vi "Configure Channel (DI Normal).vi"(0 "VISA resource name":refnum<visa-resource-name>, 5 "Channel (0001)":string="0001", 7 "Enable Channel (True)":bool=TRUE, 9 "Span":T1={"Lower Span (0)"=0, "Upper Span (1)"=1} {"Upper Span (1)" min=-99999 max=99999 step=1; "Lower Span (0)" min=-99999 max=99999 step=1}, 11 "error in (no error)":errorcluster) -> (4 "VISA resource name out":refnum<visa-resource-name>, 6 "Channel":string, 15 "error out":errorcluster)   [LabVIEW 2020, in "Yokogawa GX Series.lvlib"]
doc: "Sets the input range of DI channels.\n\nCommand: SRangeDI"
uses:
  <instrlib>/Yokogawa GX Series/Yokogawa GX Series.lvlib
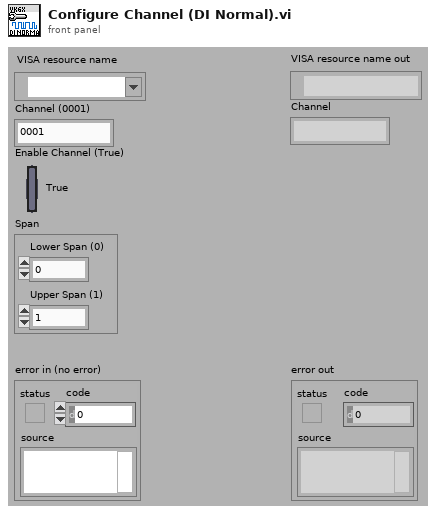
[diagram p1: front panel]
types:
  T1 = cluster{"Lower Span (0)":i32, "Upper Span (1)":i32}
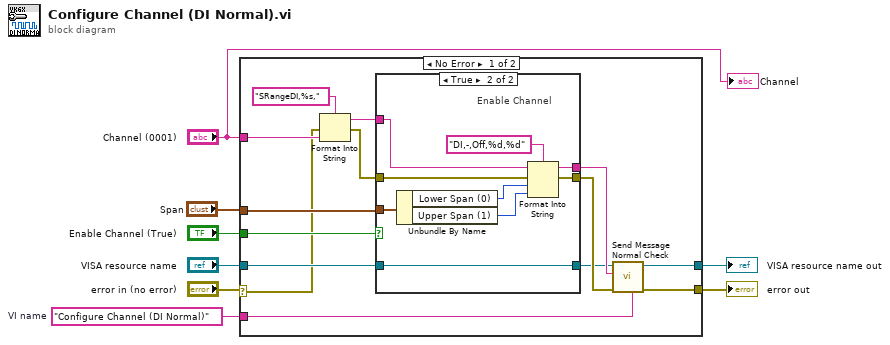
[diagram p0: block diagram]
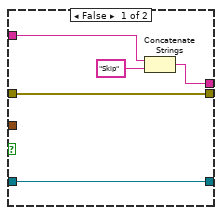
[diagram p2: hidden frame]
diagram:
  w5 = "Configure Channel (DI Normal)"  # VI name
  n1 = case shown="No Error" "error in (no error)" {
    selector: "error in (no error)" -> [w9 w37]
    tunnel: "Enable Channel (True)" -> [w19 _]
    tunnel: [w18 w38] -> w7
    tunnel: [w17 w37] -> w6
    tunnel: w5 -> [w14 _]
    tunnel: "Span" -> [w13 _]
    tunnel: "VISA resource name" -> [w12 w38]
    tunnel: "Channel (0001)" -> [w10 _]
    frame No Error {
      n2 = Format Into String(format string="SRangeDI,%s,", error in=w9, w10) -> (resulting string=w20:string, error out=w21:errorcluster)  [unwired: 1 in]
      n3 = case shown="True" w19 {
        tunnel: w21 -> [w24 w35]
        tunnel: [w24 w34] -> w16
        tunnel: w20 -> [w25 w28]
        tunnel: [w26 w33] -> w15
        tunnel: w13 -> [_ w32]
        tunnel: w12 -> [w23 w31]
        tunnel: [w23 w31] -> w11
        frame False {
          n4 = Concatenate Strings(w25, "Skip") -> (w26:string)
        }
        frame True {
          # "Enable Channel"
          n5 = Unbundle By Name(w32) -> ("Lower Span (0)"=w30:i32, "Upper Span (1)"=w29:i32)
          n6 = Format Into String(format string="DI,-,Off,%d,%d", initial string=w28, error in=w35, w30, w29) -> (resulting string=w33:string, error out=w34:errorcluster)
        }
      }
      n7 = call <instrlib>:"Send Message Normal Check.vi"("Source (\"\")"=w14, "error in (no error)"=w16, "Send Message (\"\")"=w15, "VISA resource name"=w11) -> ("error out"=w17:errorcluster, "VISA resource name out"=w18:refnum<visa-resource-name>)  [unwired: 2 in, 4 out]
    }
    frame Error {
    }
  }
  "error out" <- w6
  "VISA resource name out" <- w7
  "Channel" <- "Channel (0001)"
